vi "waitForTrav.vi"(8 "error in":errorcluster) -> (0 "error out":errorcluster)   [LabVIEW 2017]
panel:
  out "Traverse is moving?":bool
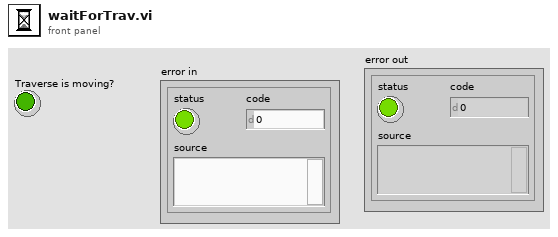
[diagram p1: front panel]
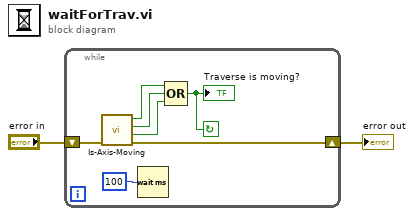
[diagram p0: block diagram]
diagram:
  n1 = while {
    shift-right: [w3] -> w1
    shift-left: "error in" -> [w4]
    stop <- w5 continue-if-true
    n2 = call "Is-Axis-Moving.vi"("error in"=w4) -> ("error out"=w3:errorcluster, "Z"=w6:bool, "Y"=w7:bool, "X"=w8:bool)  [unwired: 7 in]
    n3 = Wait (ms)(milliseconds to wait=u32 100) -> ()  [unwired: 1 out]
    n4 = Compound Arithmetic op=OR(w8, w7, w6) -> (w5:bool)
    "Traverse is moving?" <- w5
  }
  "error out" <- w1
